vi "Next Interval.vi"(10 "Interval Token in":T1, 11 "Intervals in":T2[](array[typedef])) -> (1 "Next interval time (ms)":u32, 2 "Interval Token out":T1, 3 "Intervals out":T2[](array[typedef]))   [LabVIEW 2021, in "Interval Timer.lvlib"]
uses:
  Interval Timer.lvlib
  Repeat Interval.ctl
  Interval Length.ctl
  Interval Token.ctl
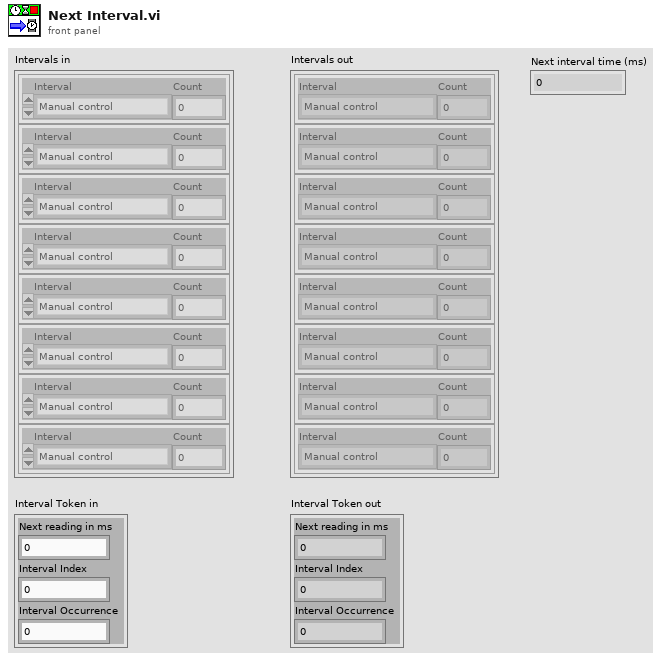
[diagram p1: front panel]
types:
  T1 = typedef "Interval Timer.lvlib/Interval Token.ctl" = cluster{"Next reading in ms":u32, "Interval Index":i32, "Interval Occurrence":i32}
  T2 = typedef "Interval Timer.lvlib/Repeat Interval.ctl" = cluster{"Interval":T3, "Count":i32}
  T3 = typedef "Interval Timer.lvlib/Interval Length.ctl" = enum16{"Manual control", "1 second", "10 seconds", "30 seconds", "60 seconds", "600 seconds", "1200 seconds", "3600 seconds"}
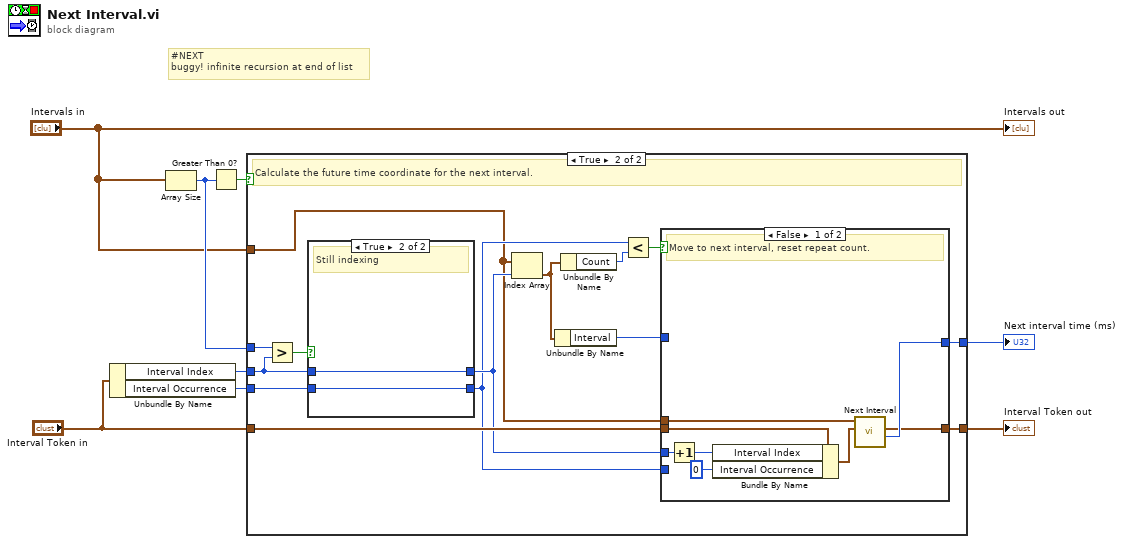
[diagram p0: block diagram]
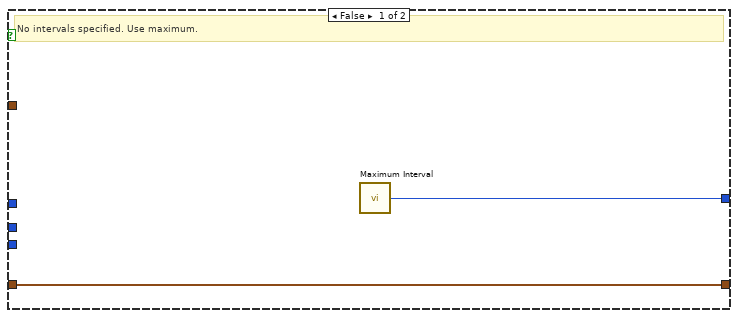
[diagram p2: hidden frame]
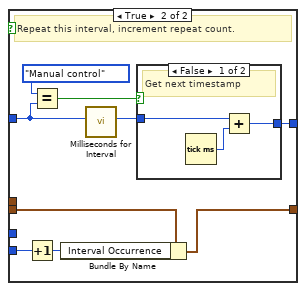
[diagram p3: hidden frame]
diagram:
  # "#NEXT\nbuggy! infinite recursion at end of list"
  n1 = Unbundle By Name("Interval Token in") -> ("Interval Index"=w6:i32, "Interval Occurrence"=w7:i32)
  n2 = Array Size(array="Intervals in") -> (size(s)=w8:i32)
  n3 = Greater Than 0?(x=w8) -> (x > 0?=w1:bool)
  n4 = case shown="True" w1 {
    tunnel: w8 -> [_ w23]
    tunnel: w7 -> [_ w22]
    tunnel: w6 -> [_ w21]
    tunnel: "Interval Token in" -> [w10 w19]
    tunnel: [w9 w15] -> w4
    tunnel: [w10 w14] -> w3
    tunnel: "Intervals in" -> [_ w11]
    frame False {
      # "No intervals specified. Use maximum."
      n5 = call "Maximum Interval.vi"() -> ("New Acquisition Time"=w9:u32)
    }
    frame True {
      # "Calculate the future time coordinate for the next interval."
      n6 = Greater?(x=w23, y=w21) -> (0:w24:bool)
      n7 = case shown="True" w24 {
        tunnel: w22 -> [w47 w48]
        tunnel: [w46 w49] -> w18
        tunnel: [w47 w48] -> w16
        tunnel: w21 -> [w46 w49]
        frame False {
          # "End of list"
        }
        frame True {
          # "Still indexing"
        }
      }
      n8 = Index Array(array=w11, index=w18) -> (element=w12:T2)
      n9 = Unbundle By Name(w12) -> ("Interval"=w17:T3)
      n10 = Unbundle By Name(w12) -> ("Count"=w13:i32)
      n11 = Less?(x=w16, y=w13) -> (x < y?=w20:bool)
      n12 = case shown="False" w20 {
        tunnel: w19 -> [w32 w41]
        tunnel: w18 -> [w30 _]
        tunnel: w17 -> [_ w36]
        tunnel: w16 -> [_ w39]
        tunnel: [w28 w38] -> w15
        tunnel: [w26 w34] -> w14
        tunnel: w11 -> [w25 _]
        frame False {
          # "Move to next interval, reset repeat count."
          n13 = Increment(x=w30) -> (x+1=w31:i32)
          n14 = Bundle By Name(cluster=w32, "Interval Index"=w31, "Interval Occurrence"=0) -> (w27:T1)
          n15 = call "Next Interval.vi"("Interval Token in"=w27, "Intervals in"=w25) -> ("Next interval time (ms)"=w28:u32, "Interval Token out"=w26:T1)  [unwired: 7 in, 1 out]
        }
        frame True {
          # "Repeat this interval, increment repeat count."
          n16 = Increment(x=w39) -> (x+1=w40:i32)
          n17 = Equal?(x=Interval_Length."Manual control" ("Interval"), y=w36) -> (x = y?=w37:bool)
          n18 = Bundle By Name(cluster=w41, "Interval Occurrence"=w40) -> (w34:T1)
          n19 = call "Milliseconds for Interval.vi"("Interval"=w36) -> ("Milliseconds"=w35:u32)  [unwired: 10 in]
          n20 = case shown="False" w37 {
            tunnel: [w43 w45] -> w38
            tunnel: w35 -> [w42 w45]
            frame False {
              # "Get next timestamp"
              n21 = Tick Count (ms)() -> (millisecond timer value=w44:u32)
              n22 = Add(x=w42, y=w44) -> (x+y=w43:u32)
            }
            frame True {
              # "Use special-case value"
            }
          }
        }
      }
    }
  }
  "Next interval time (ms)" <- w4
  "Interval Token out" <- w3
  "Intervals out" <- "Intervals in"
